vi "update camera op mode error.vi"(8 "error in (no error)":errorcluster, 11 "Channel in":refnum<class "Channel.lvclass">) -> (0 "error out":errorcluster, 3 "Channel out":refnum<class "Channel.lvclass">)   [LabVIEW 2018, in "Channel.lvclass"]
doc: "Verify if there is an error in the error array of the camera class\n\nThis function will return true if there is any error or warning in the error array of the camera with a code different of 20002 or 0."
uses:
  Channel.lvclass
  Channel.lvclass/Channel.ctl
  <vilib>/Utility/error.llb/Error Cluster From Error Code.vi
  <vilib>/ErrorRing/Error Ring.xnode
  Simulated_CCD_Camera/Simulated Camera.lvclass
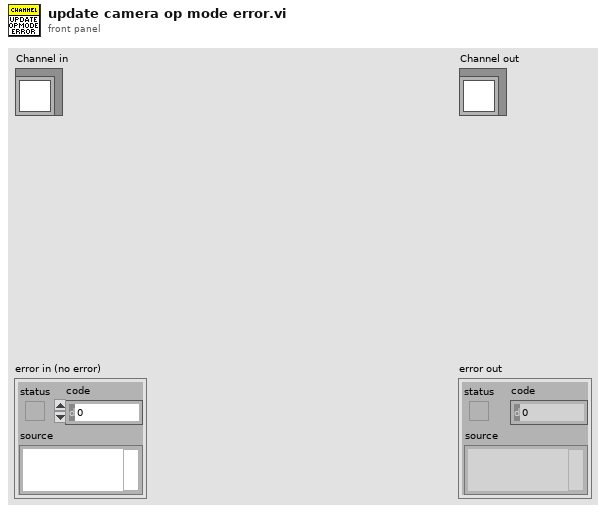
[diagram p1: front panel]
types:
  T1 = cluster{"CYCLES_DONE":u16, "LAST_IMAGE_NAME":string, "USED_DISK_SPACE":u16, "FRAMES_DONE":u16, "CCD_STATUS":string, "CURRENT_TEMPERATURE":i16, "TEMPERATURE_STATUS":string, "FRAME_EXPOSURE_TIME":sgl, "ERROR":bool, "SERIAL_NUMBER":u16, "ACQUIRING":bool, "IMAGE_INDEX":u32, "SEQS_DONE":u16}
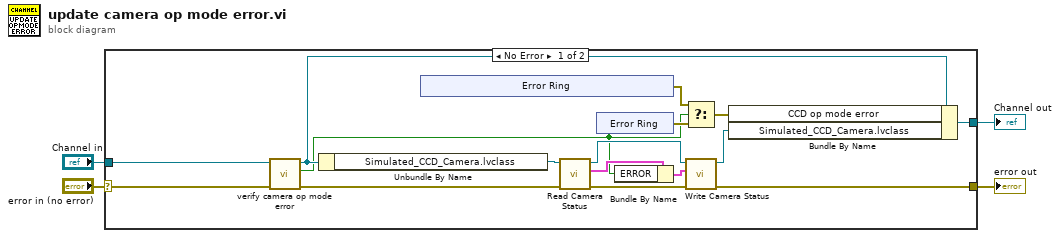
[diagram p0: block diagram]
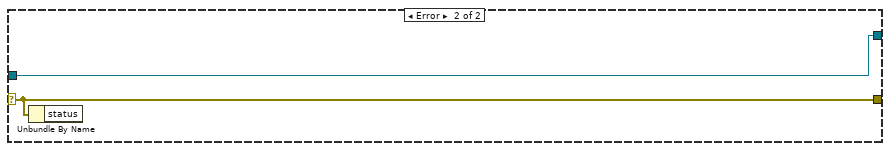
[diagram p2: hidden frame]
diagram:
  n1 = case shown="No Error" "error in (no error)" {
    selector: "error in (no error)" -> [w7 w27]
    tunnel: [w14 w27] -> w3
    tunnel: [w20 w28] -> w1
    tunnel: "Channel in" -> [w9 w28]
    frame No Error {
      n2 = call "verify camera op mode error.vi"("error in (no error)"=w7, "Channel in"=w9) -> ("error out"=w8:errorcluster, "logical OR"=w5:bool, "Channel out"=w6:refnum<class "Channel.lvclass">)  [unwired: 7 in]
      n3 = Unbundle By Name(w6) -> ("Simulated_CCD_Camera.lvclass"=w10:refnum<class "Simulated Camera.lvclass">)
      n4 = xnode "Error Ring"() -> ("error out"=w19:errorcluster)
      n5 = call "Read Camera Status.vi"("error in (no error)"=w8, "CCDCamera in"=w10) -> ("error out"=w13:errorcluster, "Camera Status"=w12:T1, "CCDCamera out"=w16:refnum<class "Simulated Camera.lvclass">)  [unwired: 7 in]
      n6 = xnode "Error Ring"() -> ("error out"=w17:errorcluster)
      n7 = Bundle By Name(cluster=w12, "ERROR"=w5) -> (w11:T1)
      n8 = Select(t=w19, s=w5, f=w17) -> (s? t:f=w18:errorcluster)
      n9 = call "Write Camera Status.vi"("error in (no error)"=w13, "Camera Status"=w11, "CCDCamera in"=w16) -> ("error out"=w14:errorcluster, "CCDCamera out"=w15:refnum<class "Simulated Camera.lvclass">)  [unwired: 7 in]
      n10 = Bundle By Name(cluster=w6, "CCD op mode error"=w18, "Simulated_CCD_Camera.lvclass"=w15) -> (w20:refnum<class "Channel.lvclass">)
    }
    frame Error {
      n11 = Unbundle By Name(w27) -> ()  [unwired: 1 out]
    }
  }
  "error out" <- w3
  "Channel out" <- w1
